vi "run_protocol_setpoint.vi"() -> ()   [LabVIEW 2011]
uses:
  protocol_Generic/Protocol_Generic.lvclass
  protocol_A/Protocol_a.lvclass
  protocol_B/Protocol_B.lvclass
  protocol_MoveToSetpoint/Protocol_MoveToSetpoint.lvclass
panel:
  in  "moveToSetpoint_setPoint":dbl
  in  "moveToSetpoint_setPointTime":dbl=5.0
  in  "Protocol":enum16{"generic", "a", "b", "move to setpoint"}(ring)
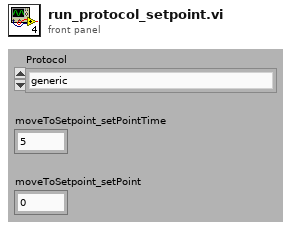
[diagram p1: front panel]
types:
  T1 = cluster{"Axis Information":cluster{"Device ID":i32, "Device Name":string, "Device Type":i32}[], "Axis Selector":i32[], "Control Modes out":u16[], "error out":errorcluster, "Channel Data":cluster{"Name":string, "Type":i32, "SI Full Scale":dbl, "Full Scale":dbl, "Units String":string, "Display Format":string, "Gauge Length":dbl}[][]}
  T2 = cluster{"Name":string, "Type":i32, "SI Full Scale":dbl, "Full Scale":dbl, "Units String":string, "Display Format":string, "Gauge Length":dbl}[][]
  T3 = cluster{"Device ID":i32, "Device Name":string, "Device Type":i32}[]
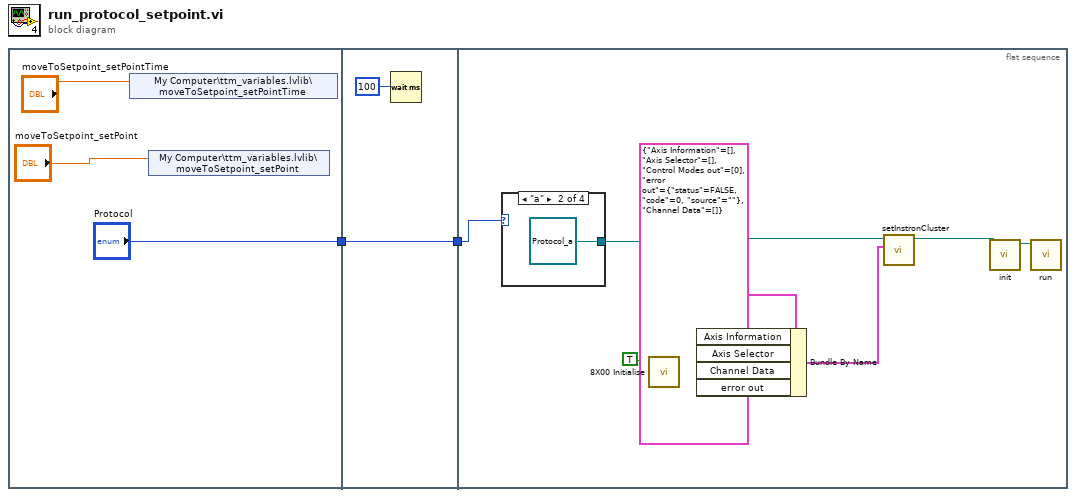
[diagram p0: block diagram]
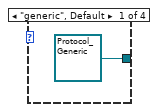
[diagram p2: hidden frame]
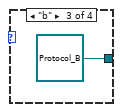
[diagram p3: hidden frame]
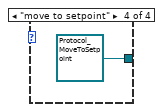
[diagram p4: hidden frame]
diagram:
  n1 = flat-sequence {
    tunnel: ["Protocol"] -> w1
    tunnel: [w6] -> w2
    tunnel: w1 -> [w6]
    tunnel: w2 -> [w18]
    frame #0 {
      n2 = shared-variable "My Computer\\ttm_variables.lvlib\\moveToSetpoint_setPointTime"("moveToSetpoint_setPointTime") -> ()  [unwired: 1 in, 1 out]
      n3 = shared-variable "My Computer\\ttm_variables.lvlib\\moveToSetpoint_setPoint"("moveToSetpoint_setPoint") -> ()  [unwired: 1 in, 1 out]
    }
    frame #1 {
      n4 = Wait (ms)(milliseconds to wait=u32 100) -> ()  [unwired: 1 out]
    }
    frame #2 {
      w15 = TRUE ("Create Console? (T)")
      n5 = case shown="\"a\"" w18 {
        tunnel: [refnum<class "Protocol_Generic.lvclass"> refnum ("Protocol_Generic.lvclass") refnum<class "Protocol_a.lvclass"> refnum ("Protocol_a.lvclass") refnum<class "Protocol_B.lvclass"> refnum ("Protocol_B.lvclass") refnum<class "Protocol_MoveToSetpoint.lvclass"> refnum ("Protocol_MoveToSetpoint.lvclass")] -> w17
        frame "generic", Default {
        }
        frame "a" {
        }
        frame "b" {
        }
        frame "move to setpoint" {
        }
      }
      n6 = call "8X00 Initialise.vi"("Reset?"=w15, "Create DVM? (T)"=w15, "Create Console? (T)"=w15) -> ("error out"=w10:errorcluster, "Channel Data"=w9:T2, "Axis Selector"=w11:i32[], "Axis Information"=w12:T3)  [unwired: 1 in]
      n7 = Bundle By Name(cluster=T1 {"Axis Information"=[], "Axis Selector"=[], "Control Modes out"=[0], "error out"={"status"=FALSE, "code"=0, "source"=""}, "Channel Data"=[]} ("InstronCluster"), "Axis Information"=w12, "Axis Selector"=w11, "Channel Data"=w9, "error out"=w10) -> (w13:T1)
      n8 = call-dynamic "setInstronCluster.vi"("InstronCluster"=w13, "Protocol_Generic in"=w17) -> ("Protocol_Generic out"=w14:refnum<class "Protocol_Generic.lvclass">)  [unwired: 8 in, 1 out]
      n9 = call-dynamic "init.vi"("Protocol_Generic in"=w14) -> ("Protocol_Generic out"=w16:refnum<class "Protocol_Generic.lvclass">)  [unwired: 9 in, 1 out]
      n10 = call-dynamic "run.vi"("Protocol_Generic in"=w16) -> ()  [unwired: 9 in, 2 out]
    }
  }
